vi "Get RTDriver Info.vi"(8 "error in (no error)":errorcluster) -> (0 "error out":errorcluster, 1 "RT Driver Info":T1[](array[typedef]))   [LabVIEW 2019, in "TemplatePPL System Explorer.lvlib"]
uses:
  TemplatePPL System Explorer.lvlib
  <vilib>/NI/NI VeriStand Advanced SysDef API/_Types/Property.DependentFile.ctl
  <vilib>/Utility/LVLibp/NI_PackedLibraryUtility.lvlib
  <vilib>/NI/NI VeriStand Advanced SysDef API/SysDef API/Advanced System Definition.lvlib
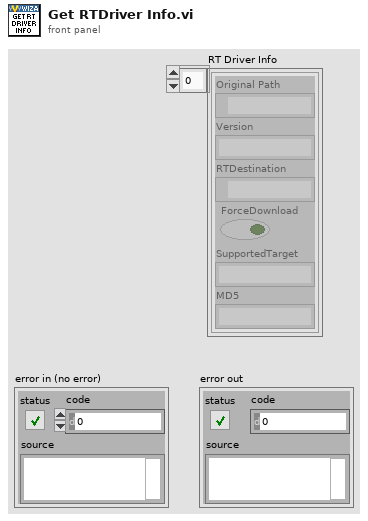
[diagram p1: front panel]
types:
  T1 = typedef "Advanced System Definition.lvlib/Property.DependentFile.ctl" = cluster{"Original Path":path, "Version":string, "RTDestination":path, "ForceDownload":bool, "SupportedTarget":string, "MD5":string}
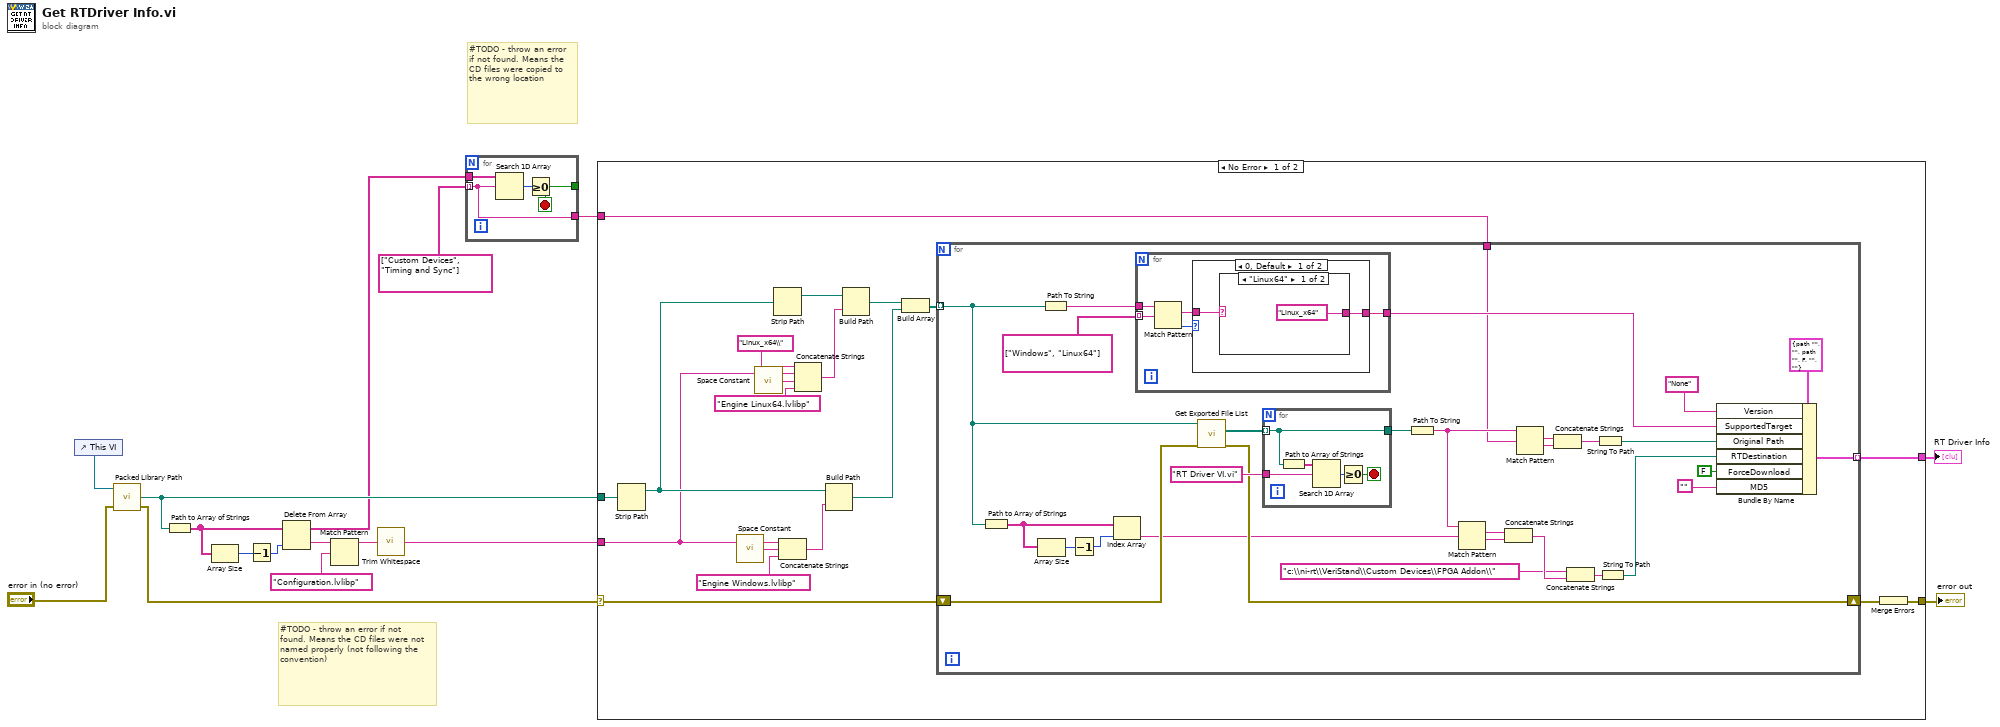
[diagram p0: block diagram]
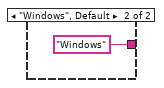
[diagram p2: hidden frame]
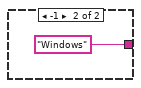
[diagram p3: hidden frame]
diagram:
  # "#TODO - throw an error if not found. Means the CD files were not named properly (not following the convention)"
  # "#TODO - throw an error if not found. Means the CD files were copied to the wrong location"
  n1 = control-ref of="This VI"() -> (w14:refnum<vi>)
  n2 = call <vilib>:"Packed Library Path.vi"("error in (no error)"="error in (no error)", "vi reference"=w14) -> ("error out"=w13:errorcluster, "packed library path"=w11:path)  [unwired: 1 in, 1 out]
  n3 = Path to Array of Strings(0:w11) -> (2:w10:string[])  [unwired: 1 out]
  n4 = Array Size(array=w10) -> (size(s)=w9:i32)
  n5 = Decrement(x=w9) -> (x-1=w8:i32)
  n6 = Delete From Array(array=w10, index=w8) -> (deleted portion=w7:string, array with subset deleted=w3:string[])  [unwired: 1 in]
  n7 = Match Pattern(string=w7, regular expression="Configuration.lvlibp") -> (before substring=w1:string)  [unwired: 1 in, 3 out]
  n8 = call <vilib>:"Trim Whitespace.vi"("string"=w1) -> ("trimmed string"=w5:string)  [unwired: 1 in]
  n9 = for {
    tunnel: string[] ["Custom Devices", "Timing and Sync"] ("array of strings") -> [w17] mode=indexing
    tunnel: [w19] -> _
    tunnel: w3 -> [w18]
    tunnel: [w17] -> w2
    stop <- w19 stop-if-true
    n10 = Search 1D Array(1D array=w18, element=w17) -> (index of element=w20:i32)  [unwired: 1 in]
    n11 = Greater Or Equal To 0?(x=w20) -> (x >= 0?=w19:bool)
  }
  n12 = case shown="No Error" w13 {
    selector: w13 -> [w31 w85]
    tunnel: w11 -> [w34 _]
    tunnel: [w30 w85] -> w15
    tunnel: [w33 _] -> w12
    tunnel: w5 -> [w25 _]
    tunnel: w2 -> [w21 _]
    frame No Error {
      n13 = Strip Path(path=w34) -> (stripped path=w36:path)  [unwired: 1 out]
      n14 = call <vilib>:"Space Constant.vi"() -> ("String"=w24:string)
      n15 = call <vilib>:"Space Constant.vi"() -> ("String"=w28:string)
      n16 = Strip Path(path=w36) -> (stripped path=w35:path)  [unwired: 1 out]
      n17 = Concatenate Strings(w25, w24, "Engine Windows.lvlibp" ("string")) -> (w22:string)
      n18 = Concatenate Strings("Linux_x64\\" ("string"), w25, w28, "Engine Linux64.lvlibp" ("string")) -> (w26:string)
      n19 = Build Path(base path=w36, name or relative path=w22) -> (appended path=w38:path)
      n20 = Build Path(base path=w35, name or relative path=w26) -> (appended path=w37:path)
      n21 = Build Array(w37, w38) -> (w39:path[])
      n22 = for {
        shift-right: [w66] -> w32
        shift-left: w31 -> [w67]
        tunnel: w39 -> [w47] mode=indexing
        tunnel: [w42] -> w33 mode=indexing
        tunnel: w21 -> [w41]
        n23 = Path to Array of Strings(0:w47) -> (2:w55:string[])  [unwired: 1 out]
        n24 = Array Size(array=w55) -> (size(s)=w57:i32)
        n25 = Path To String(path=w47) -> (string=w46:string)
        n26 = Decrement(x=w57) -> (x-1=w56:i32)
        n27 = Index Array(array=w55, index=w56) -> (element=w54:string)
        n28 = for {
          tunnel: w46 -> [w74]
          tunnel: string[] ["Windows", "Linux64"] -> [w73] mode=indexing
          tunnel: [w70] -> w44
          n29 = Match Pattern(string=w74, regular expression=w73) -> (match substring=w71:string, offset past match=w72:i32)  [unwired: 1 in, 2 out]
          n30 = case shown="0, Default" w72 {
            tunnel: w71 -> [w76 _]
            tunnel: [w75 "Windows" ("regular expression")] -> w70
            frame 0, Default {
              n31 = case shown="\"Linux64\"" w76 {
                tunnel: ["Linux_x64" ("regular expression") "Windows" ("regular expression")] -> w75
                frame "Linux64" {
                }
                frame "Windows", Default {
                }
              }
            }
            frame -1 {
            }
          }
        }
        n32 = call <vilib>:"Get Exported File List.vi"("error in (no error)"=w67, "packed library path"=w47) -> ("error out"=w66:errorcluster, "paths"=w69:path[])  [unwired: 7 in, 1 out]
        n33 = for {
          tunnel: w69 -> [w81] mode=indexing
          tunnel: "RT Driver VI.vi" ("element") -> [w83]
          tunnel: [w81] -> w65
          stop <- w80 stop-if-true
          n34 = Path to Array of Strings(0:w81) -> (2:w84:string[])  [unwired: 1 out]
          n35 = Search 1D Array(1D array=w84, element=w83) -> (index of element=w82:i32)  [unwired: 1 in]
          n36 = Greater Or Equal To 0?(x=w82) -> (x >= 0?=w80:bool)
        }
        n37 = Path To String(path=w65) -> (string=w62:string)
        n38 = Match Pattern(string=w62, regular expression=w54) -> (match substring=w61:string, after substring=w60:string)  [unwired: 1 in, 2 out]
        n39 = Concatenate Strings(w61, w60) -> (w59:string)
        n40 = Match Pattern(string=w62, regular expression=w41) -> (match substring=w64:string, after substring=w63:string)  [unwired: 1 in, 2 out]
        n41 = Concatenate Strings(w64, w63) -> (w52:string)
        n42 = Concatenate Strings("c:\\ni-rt\\VeriStand\\Custom Devices\\FPGA Addon\\" ("regular expression"), w59) -> (w50:string)
        n43 = String To Path(string=w52) -> (path=w51:path)
        n44 = String To Path(string=w50) -> (path=w49:path)
        n45 = Bundle By Name(cluster=T1 {"Original Path"=path "", "Version"="", "RTDestination"=path "", "ForceDownload"=FALSE, "SupportedTarget"="", "MD5"=""} ("OptionalInfo"), "Version"="None", "SupportedTarget"=w44, "Original Path"=w51, "RTDestination"=w49, "ForceDownload"=FALSE, "MD5"="") -> (w42:T1)
      }
      n46 = Merge Errors(w32) -> (w30:errorcluster)
    }
    frame Error {
    }
  }
  "error out" <- w15
  "RT Driver Info" <- w12
